vi "SL TAGS Class Type To SystemLink.vi"(8 "error in (no error)":errorcluster, 11 "Class Tag In":T1={"Class Properties"={"Class Data Type"=enum."Double", "Name"="", "Description"="", "Interpolation Method"=enum."linear", "Unit of Measure"=enum."Hour", "Maximum Interpolation"="", "Role"=enum."Supervisor"}, "SL Tag"=refnum, "SystemLink Cluster"={"Path"="", "Data Type"=enum."Double", "Value"=variant, "Time Stamp"=timestamp(0 s since 1904-01-01)}, "Class Value"=variant}) -> (0 "error out":errorcluster, 2 "SL Tag":refnum<class "NI Skyline Tag.lvclass">, 3 "Class Tag Out":T1={"Class Properties"={"Class Data Type"=enum."Double", "Name"="", "Description"="", "Interpolation Method"=enum."linear", "Unit of Measure"=enum."Hour", "Maximum Interpolation"="", "Role"=enum."Supervisor"}, "SL Tag"=refnum, "SystemLink Cluster"={"Path"="", "Data Type"=enum."Double", "Value"=variant, "Time Stamp"=timestamp(0 s since 1904-01-01)}, "Class Value"=variant})   [LabVIEW 2017, in "EEISysLink.lvclass"]
doc: "At time of this library development SystemLink has mixed or no support for booleans & waveforms. This VI translates an extended set of data types in the class and more restricted in the SystemLink server from class type to SystemLink type.\n\nIt takes the input class value and updates the value in the SystemLink Cluster. \n\nThis is a good location to seperate data types in SystemLink from those in the class. This allows the class to support any number of data types and translate to SystemLink types. This class translation is a good candidate for extending with additional data type classes to support an extended library functionality. \n\nJames Tillett P.E.\nEndeavor Engineering Inc.\nwww.endeavoreng.com"
uses:
  EEISysLink.lvclass
  Controls/SL Tag.ctl
  <vilib>/Skyline/Tag/Wrapper/Wrapper_class/NI Skyline Tag.lvclass
  Controls/SL Tag Properties.ctl
  Controls/SL Tag Data Type.ctl
  Controls/SL Tag Interpolation Method.ctl
  Controls/SL Tag Unit of Measure.ctl
  Controls/SL Tag Type.ctl
  <vilib>/Skyline/Tag/Shared/typedefs/Tag Cluster.ctl
  <vilib>/Skyline/Tag/Shared/typedefs/DataType.ctl
  Controls/SL Waveform.ctl
  <vilib>/Skyline/Tag/Shared/NI Skyline Tag.lvlib
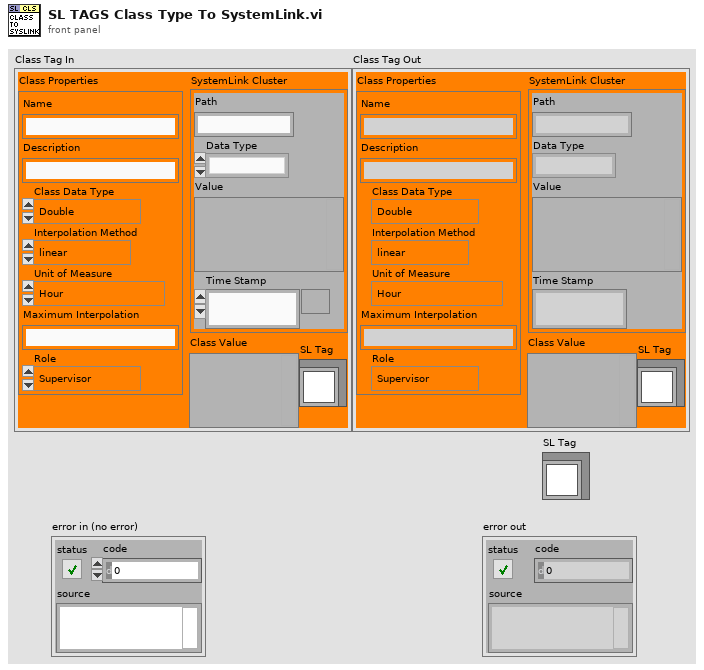
[diagram p1: front panel]
types:
  T1 = typedef "EEISysLink.lvclass/SL Tag.ctl" = cluster{"Class Properties":T2, "SL Tag":refnum<class "NI Skyline Tag.lvclass">, "SystemLink Cluster":T7, "Class Value":variant}
  T2 = typedef "EEISysLink.lvclass/SL Tag Properties.ctl" = cluster{"Class Data Type":T3, "Name":string, "Description":string, "Interpolation Method":T4, "Unit of Measure":T5, "Maximum Interpolation":string, "Role":T6}
  T3 = typedef "EEISysLink.lvclass/SL Tag Data Type.ctl" = enum16{"Double", "Integer", "String", "Boolean", "Waveform"}
  T4 = typedef "EEISysLink.lvclass/SL Tag Interpolation Method.ctl" = enum16{"linear", "pilinear", "step"}
  T5 = typedef "EEISysLink.lvclass/SL Tag Unit of Measure.ctl" = enum16{"no units", "Second", "Hour", "Minute", "Day", "Year", "Month", "Week", "Foot", "Yard", "Meter", "Centimeter", "Inch", "Mile", "Nautical Mile", "Miles per Hour", "Meters per second", "Square meter", "Cubic meter", "Cubic centimeter", "Cubic inch", "Liter", "Gallon", "Gallons dry US", "Gallon UK", "Percent", "Revolutions per minute", "Revolution", "Degree angle", "Astronomical Unit", "Atom", "Atomic mass", "Bar", "Byte", "C (speed of light)", "Curie", "Decibel", "Electron Volt", "Ounce", "Knot", "G", "Grade", "Are", "Hectare", "Faraday", "Franklin", "Gilbert", "Erg", "Lambert", "Maxwell", "Gauss", "Electron mass", "Kilogram force", "Pound force", "Rad", "Centiradian", "Sphere", "Mach", "Fluid Ounces", "Fluid Ounces UK", "Fahrenheit", "Celsius", "Kelvin", "Rankine", "Gram", "Kilogram", "Pound", "Short/US Ton", "Long/UK ton", "Metric ton", "Mole", "Pounds per square inch", "Inches water column", "Torr", "Millitorr", "Millimeter mercury", "Inches mercury", "Bar (2)", "Atmosphere", "Pascal", "Watt", "kiloWatt", "Horsepower", "Kilowatt Hour", "British thermal units", "Millions of BTU", "Ampere", "Candela", "Radian", "Steradian", "Bit", "Hertz", "Newton", "Joule", "Coulomb", "Volt", "Farad", "Ohm", "Siemens", "Weber", "Tesla", "Henry", "Lumen", "Lux", "Becqueral", "Gray", "Sievert", "Katal", "Angstrom", "Light Year", "Parsec", "Point", "Pixel", "Dyne", "Kilogram force (2)", "Pound force (2)", "Rem", "Rutherford", "Roentgen"}
  T6 = typedef "EEISysLink.lvclass/SL Tag Type.ctl" = enum16{"All", "Supervisor", "Worker"}
  T7 = typedef "NI Skyline Tag.lvlib/Tag Cluster.ctl" = cluster{"Path":string, "Data Type":T8, "Value":variant, "Time Stamp":timestamp}
  T8 = typedef "NI Skyline Tag.lvlib/DataType.ctl" = enum32{"Double", "Integer", "String"}
  T9 = typedef "EEISysLink.lvclass/SL Waveform.ctl" = cluster{"t0":dbl, "dt":dbl, "Y":dbl[]}
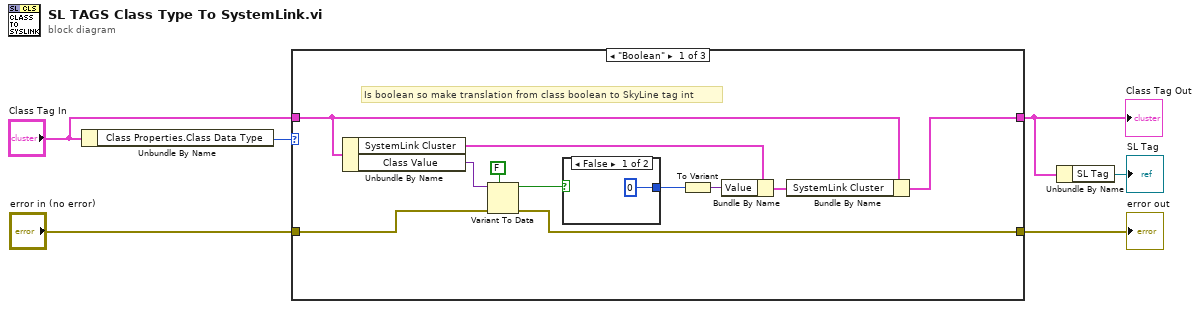
[diagram p0: block diagram]
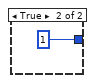
[diagram p2: hidden frame]
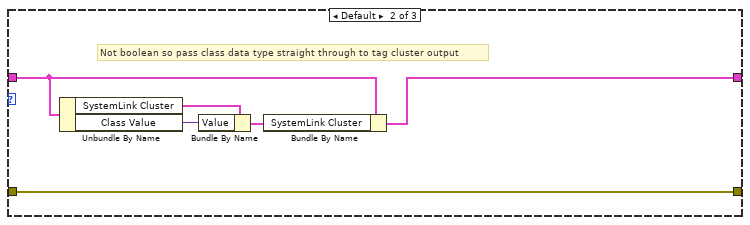
[diagram p3: hidden frame]
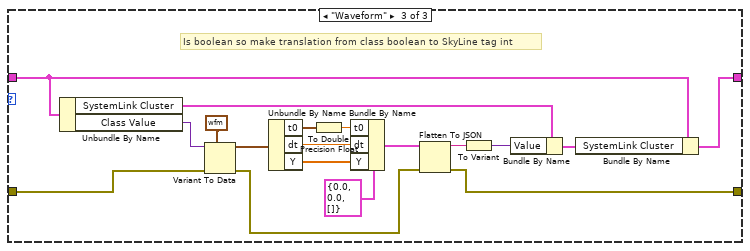
[diagram p4: hidden frame]
diagram:
  n1 = Unbundle By Name("Class Tag In") -> ("Class Properties.Class Data Type"=w6:T3)
  n2 = case shown="\"Boolean\"" w6 {
    tunnel: "Class Tag In" -> [w16 w24 w42]
    tunnel: [w15 w23 w41] -> w4
    tunnel: [w9 w20 w35] -> w3
    tunnel: "error in (no error)" -> [w13 w20 w39]
    frame "Boolean" {
      # "Is boolean so make translation from class boolean to SkyLine tag int"
      n3 = Unbundle By Name(w16) -> ("SystemLink Cluster"=w17:T7, "Class Value"=w14:variant)
      n4 = Variant To Data(error in=w13, type=FALSE, Variant=w14) -> (data=w8:bool, error out=w9:errorcluster)
      n5 = case shown="False" w8 {
        tunnel: [0 1] -> w7
        frame False {
        }
        frame True {
        }
      }
      n6 = To Variant(anything=w7) -> (Variant=w11:variant)
      n7 = Bundle By Name(cluster=w17, "Value"=w11) -> (w10:T7)
      n8 = Bundle By Name(cluster=w16, "SystemLink Cluster"=w10) -> (w15:T1)
    }
    frame Default {
      # "Not boolean so pass class data type straight through to tag cluster output"
      n9 = Unbundle By Name(w24) -> ("SystemLink Cluster"=w25:T7, "Class Value"=w21:variant)
      n10 = Bundle By Name(cluster=w25, "Value"=w21) -> (w22:T7)
      n11 = Bundle By Name(cluster=w24, "SystemLink Cluster"=w22) -> (w23:T1)
    }
    frame "Waveform" {
      # "Is boolean so make translation from class boolean to SkyLine tag int"
      n12 = Unbundle By Name(w42) -> ("SystemLink Cluster"=w43:T7, "Class Value"=w40:variant)
      n13 = Variant To Data(error in=w39, type=waveform(dbl) {"t0"=timestamp(0 s since 1904-01-01), "dt"=1.0, "Y"=[]} ("waveform in"), Variant=w40) -> (data=w33:waveform(dbl), error out=w26:errorcluster)
      n14 = Unbundle By Name(w33) -> ("t0"=w31:timestamp, "dt"=w29:dbl, "Y"=w28:dbl[])
      n15 = To Double Precision Float(number=w31) -> (double precision float=w30:dbl)
      n16 = Bundle By Name(cluster=T9 {"t0"=0.0, "dt"=0.0, "Y"=[]} ("SL Waveform"), "t0"=w30, "dt"=w29, "Y"=w28) -> (w27:T9)
      n17 = Flatten To JSON(anything=w27, error in (no error)=w26) -> (JSON string=w38:string, 11:w35:errorcluster)  [unwired: 1 in]
      n18 = To Variant(anything=w38) -> (Variant=w37:variant)
      n19 = Bundle By Name(cluster=w43, "Value"=w37) -> (w36:T7)
      n20 = Bundle By Name(cluster=w42, "SystemLink Cluster"=w36) -> (w41:T1)
    }
  }
  "Class Tag Out" <- w4
  "error out" <- w3
  n21 = Unbundle By Name(w4) -> ("SL Tag"=→"SL Tag":refnum<class "NI Skyline Tag.lvclass">)
